vi "Corr_Fact.vi"(10 "n_air":dbl, 11 "Wavelength":dbl) -> (3 "Correction Factor":dbl)   [LabVIEW 2018]
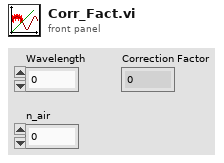
[diagram p1: front panel]
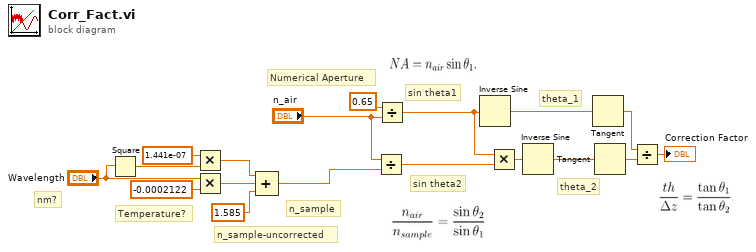
[diagram p0: block diagram]
diagram:
  # "n_sample-uncorrected"
  # "Temperature?"
  # "n_sample"
  # "sin theta2"
  # "sin theta1"
  # "nm?"
  # "Numerical Aperture"
  # "theta_2"
  # "theta_1"
  n1 = Square(x="Wavelength") -> (x^2=w11:dbl)
  n2 = Multiply(x=1.441e-07, y=w11) -> (x*y=w10:dbl)
  n3 = Multiply(x="Wavelength", y=-0.0002122 ("x")) -> (x*y=w14:dbl)
  n4 = Compound Arithmetic op=ADD(w10, w14, 1.585 ("value")) -> (w8:dbl)
  n5 = Divide(x="n_air", y=w8) -> (x/y=w9:dbl)
  n6 = Divide(x=0.65, y="n_air") -> (x/y=w4:dbl)
  n7 = Inverse Sine(1:w4) -> (0:w6:dbl)
  n8 = Multiply(x=w4, y=w9) -> (x*y=w17:dbl)
  n9 = Inverse Sine(1:w17) -> (0:w7:dbl)
  n10 = Tangent(1:w6) -> (0:w5:dbl)
  n11 = Tangent(1:w7) -> (0:w18:dbl)
  n12 = Divide(x=w5, y=w18) -> (x/y=→"Correction Factor":dbl)
